vi "IVIS FRET_Get Mask ROIs.vi"(8 "Error In":errorcluster, 9 "ROI Type List":string="DO, AO, DA", 10 "Organ":string="UB", 11 "Mask Image File":path) -> (0 "error out":errorcluster, 1 "Ordered ROI Type List":string[](array[string]), 2 "Ordered ROIs":T2[](array[typedef]) caption="ROIs" {"Contours"."Type" items=["No Selection", "Point", "Line", "Rectangle", "Oval", "Polygon", "Freehand Region", "Annulus", "Unused2", "Unused3", "Broken Line", "Freehand Line", "Rotated Rectangle"]}, 3 "Ordered Organ ROI Type Masks":T1[](array[typedef]))   [LabVIEW 2021]
uses:
  <vilib>/vision/Image Controls.llb/IMAQ Image.ctl
  <userlib>/_OpenG.lib/array/array.llb/Sort 1D Array (String)__ogtk.vi
  <userlib>/_OpenG.lib/array/array.llb/Reorder 1D Array2 (Variant)__ogtk.vi
  <vilib>/vision/NI_Vision_Development_Module.lvlib
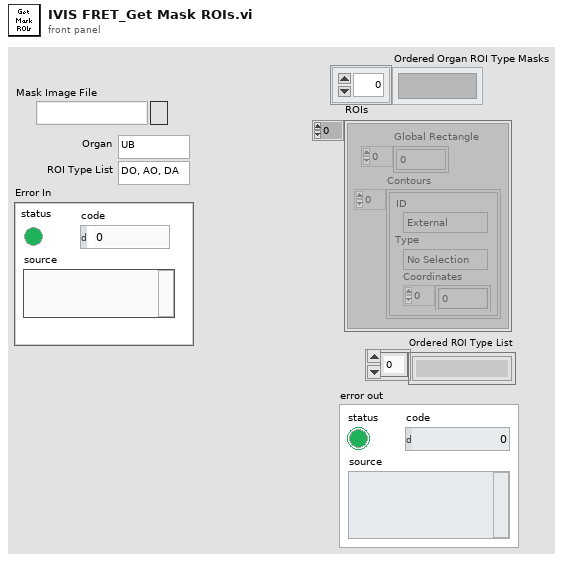
[diagram p1: front panel]
types:
  T1 = typedef "IMAQ Image.ctl" = refnum<image>
  T2 = typedef "ROI Descriptor" = cluster{"Global Rectangle":i32[], "Contours":cluster{"ID":enum32{"External", "Internal"}, "Type":u32, "Coordinates":i32[]}[]}
  T3 = typedef "Image Type" = u32
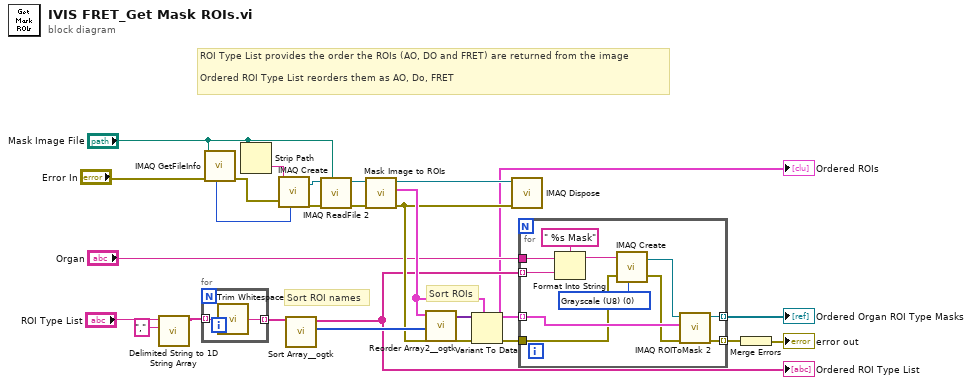
[diagram p0: block diagram]
diagram:
  # "ROI Type List provides the order the ROIs (AO, DO and FRET) are returned from the image\n\nOrdered ROI Type List reorders them as AO, Do, FRET"
  # "Sort ROIs"
  # "Sort ROI names"
  n1 = call <vilib>:"Delimited String to 1D String Array.vi"("delimiter"=",", "delimited string"="ROI Type List") -> ("string array"=w13:string[])  [unwired: 9 in]
  n2 = for {
    tunnel: w13 -> [w27] mode=indexing
    tunnel: [w26] -> w12 mode=indexing
    n3 = call <vilib>:"Trim Whitespace.vi"("string"=w27) -> ("trimmed string"=w26:string)  [unwired: 1 in]
  }
  n4 = call "IMAQ GetFileInfo"("error in (no error)"="Error In", "File Path"="Mask Image File") -> ("error out"=w24:errorcluster, "Image Type"=w22:T3)  [unwired: 3 in, 5 out]
  n5 = Strip Path(path="Mask Image File") -> (name=w19:string)  [unwired: 1 out]
  n6 = call "IMAQ Create"("Image Name"=w19, "Image Type"=w22, "error in (no error)"=w24) -> ("New Image"=w25:T1, "error out"=w21:errorcluster)  [unwired: 2 in]
  n7 = call-poly <userlib>:"Sort Array__ogtk.vi"("Array in"=w12) -> ("Sorted Pointers"=w11:i32[], "Sorted Array out"=w5:string[])  [unwired: 9 in]
  "Ordered ROI Type List" <- w5
  n8 = call "IMAQ ReadFile 2"("File Path"="Mask Image File", "error in (no error)"=w21, "Image"=w25) -> ("error out"=w17:errorcluster, "Image Out"=w18:T1)  [unwired: 4 in, 3 out]
  n9 = call "Mask Image to ROIs.vi"("Error In"=w17, "Mask Image Refnum in"=w18) -> ("Error Out"=w8:errorcluster, "ROIs"=w9:T2[], "Mask Image Refnum out"=w16:T1)  [unwired: 7 in]
  n10 = call-poly <userlib>:"Reorder Array2__ogtk.vi"("indices"=w11, "array"=w9) -> ("reordered array"=w10:variant[])  [unwired: 9 in]
  n11 = Variant To Data(error in=w8, type=w9, Variant=w10) -> (data=w1:T2[], error out=w7:errorcluster)
  "Ordered ROIs" <- w1
  n12 = call "IMAQ Dispose"("Image"=w16, "error in (no error)"=w8) -> ()  [unwired: 4 in, 1 out]
  n13 = for {
    tunnel: w1 -> [w38] mode=indexing
    tunnel: w7 -> [w31]
    tunnel: "Organ" -> [w37]
    tunnel: w5 -> [w36] mode=indexing
    tunnel: [w29] -> w3 mode=indexing
    tunnel: [w28] -> w4 mode=indexing
    w33 = T3 0 items=["Grayscale (U8)", "Grayscale (I16)", "Grayscale (SGL)", "Complex (CSG)", "RGB (U32)", "HSL (U32)", "RGB (U64)", "Grayscale (U16)"] ("Image Type")
    n14 = Format Into String(format string=" %s Mask", initial string=w37, w36) -> (resulting string=w34:string)  [unwired: 1 in, 1 out]
    n15 = call "IMAQ Create"("Image Name"=w34, "Image Type"=w33, "error in (no error)"=w31) -> ("New Image"=w30:T1, "error out"=w32:errorcluster)  [unwired: 2 in]
    n16 = call "IMAQ ROIToMask 2"("error in (no error)"=w32, "ROI Descriptor"=w38, "Image"=w30) -> ("error out"=w29:errorcluster, "Image Out"=w28:T1)  [unwired: 6 in, 1 out]
  }
  "Ordered Organ ROI Type Masks" <- w4
  n17 = Merge Errors(w3) -> (→"error out":errorcluster)
